vi "Get Image.vi"(8 "error in (no error)":errorcluster, 11 "Image Acquisition in":refnum<class "Camera.lvclass">) -> (0 "error out":errorcluster, 2 "Image Reference":T1, 3 "Image Acquisition out":refnum<class "Camera.lvclass">)   [LabVIEW 2018, in "Camera.lvclass"]
uses:
  Camera.lvclass
  <vilib>/vision/Image Controls.llb/IMAQ Image.ctl
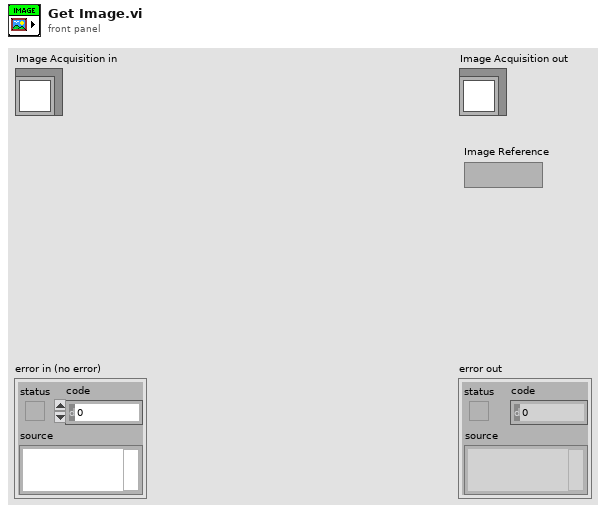
[diagram p1: front panel]
types:
  T1 = typedef "IMAQ Image.ctl" = refnum<image>
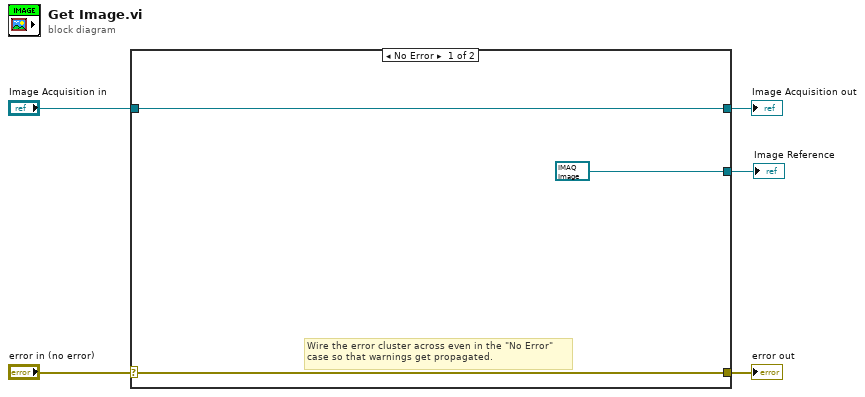
[diagram p0: block diagram]
diagram:
  n1 = case shown="No Error" "error in (no error)" {
    selector: "error in (no error)" -> [w7 w10]
    tunnel: [w7 w10] -> w4
    tunnel: [w8 w9] -> w2
    tunnel: "Image Acquisition in" -> [w8 w9]
    tunnel: [T1 refnum ("Image Out") _] -> w1
    frame No Error {
      # "Wire the error cluster across even in the \"No Error\"\ncase so that warnings get propagated."
    }
    frame Error {
    }
  }
  "error out" <- w4
  "Image Acquisition out" <- w2
  "Image Reference" <- w1
